vi "Pod Health Status.vi"(7 "Pod Health Configuration":T1={"Power"={"Batt. Current Max (A)"=400.0, " Batt. Current Min (A)"=200.0, "Batt. Voltage Min (V)"=11.5, "Batt. Voltage Max (V)"=13.0, "Brake Current Max (A)"=1.5, " Brake Current Min (A)"=1.3, "Brake Voltage Min (V)"=23.0, "Brake Voltage Max (V)"=25.0}, "Pressure"={"Tank Max (PSI)"=3000.0, "Tank Min (PSI)"=2000.0, "Utility Max (PSI)"=350.0, "Utility Min (PSI)"=250.0, "Brake Max (PSI)"=250.0, "Brake Min (PSI)"=150.0, "Levitation Max (PSI)"=55.0, "Levitation Min (PSI)"=45.0}, "Position"={"Lev. Min (mm)"=35.0, "Lev. Max (mm)"=75.0}}, 10 "Telemetry":T2 {"Brake Pressure (PSI)" scale=0.0..1000.0; "Maglock 4 (mm)" scale=0.0..15.0; "Maglock 3 (mm)" scale=0.0..15.0; "Maglock 2 (mm)" scale=0.0..15.0; "Maglock 1 (mm)" scale=0.0..15.0; "ToF 4 (mm)" scale=0.0..100.0; "ToF 3 (mm)" scale=0.0..100.0; "ToF 2 (mm)" scale=0.0..100.0; "ToF 1 (mm)" scale=0.0..100.0; "Levitation Pressure (PSI)" scale=0.0..1000.0; "Utility Pressure (PSI)" scale=0.0..1000.0; "Tank Pressure (PSI)" scale=0.0..1000.0; "Brake Voltage (V)" scale=0.0..15.0; "Battery Voltage (V)" scale=0.0..15.0; "Brake Current (A)" scale=0.0..500.0; "Battery Current (A)" scale=0.0..500.0}) -> (2 "Pod Health":T3)   [LabVIEW 2018]
uses:
  Type Defs/PodHealth.ctl
  Type Defs/prettyTelemetry.ctl
  Type Defs/PodHealthConfig.ctl
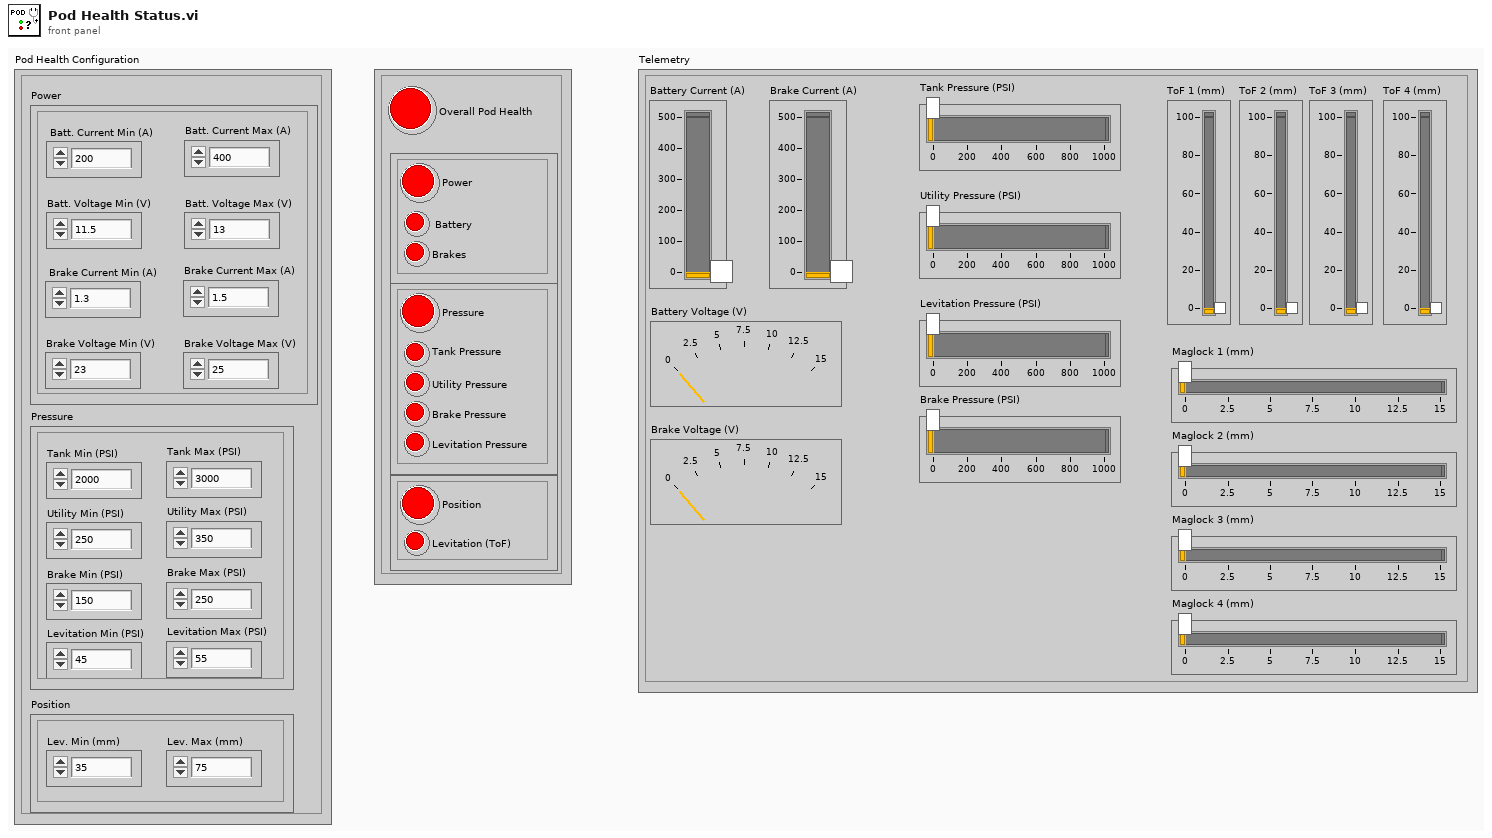
[diagram p1: front panel]
types:
  T1 = typedef "PodHealthConfig.ctl" = cluster{"Power":cluster{"Batt. Current Max (A)":dbl, " Batt. Current Min (A)":dbl, "Batt. Voltage Min (V)":dbl, "Batt. Voltage Max (V)":dbl, "Brake Current Max (A)":dbl, " Brake Current Min (A)":dbl, "Brake Voltage Min (V)":dbl, "Brake Voltage Max (V)":dbl}, "Pressure":cluster{"Tank Max (PSI)":dbl, "Tank Min (PSI)":dbl, "Utility Max (PSI)":dbl, "Utility Min (PSI)":dbl, "Brake Max (PSI)":dbl, "Brake Min (PSI)":dbl, "Levitation Max (PSI)":dbl, "Levitation Min (PSI)":dbl}, "Position":cluster{"Lev. Min (mm)":dbl, "Lev. Max (mm)":dbl}}
  T2 = typedef "prettyTelemetry.ctl" = cluster{"Battery Current (A)":dbl, "Brake Current (A)":dbl, "Battery Voltage (V)":dbl, "Brake Voltage (V)":dbl, "Tank Pressure (PSI)":dbl, "Utility Pressure (PSI)":dbl, "Levitation Pressure (PSI)":dbl, "Brake Pressure (PSI)":dbl, "ToF 1 (mm)":dbl, "ToF 2 (mm)":dbl, "ToF 3 (mm)":dbl, "ToF 4 (mm)":dbl, "Maglock 1 (mm)":dbl, "Maglock 2 (mm)":dbl, "Maglock 3 (mm)":dbl, "Maglock 4 (mm)":dbl}
  T3 = typedef "PodHealth.ctl" = cluster{"Overall Pod Health":bool, "Power":cluster{"Power":bool, " Battery":bool, "Brakes":bool}, "Pressure":cluster{"Pressure":bool, "Tank Pressure":bool, "Utility Pressure":bool, "Brake Pressure":bool, "Levitation Pressure":bool}, "Position":cluster{"Position":bool, "Levitation (ToF)":bool}}
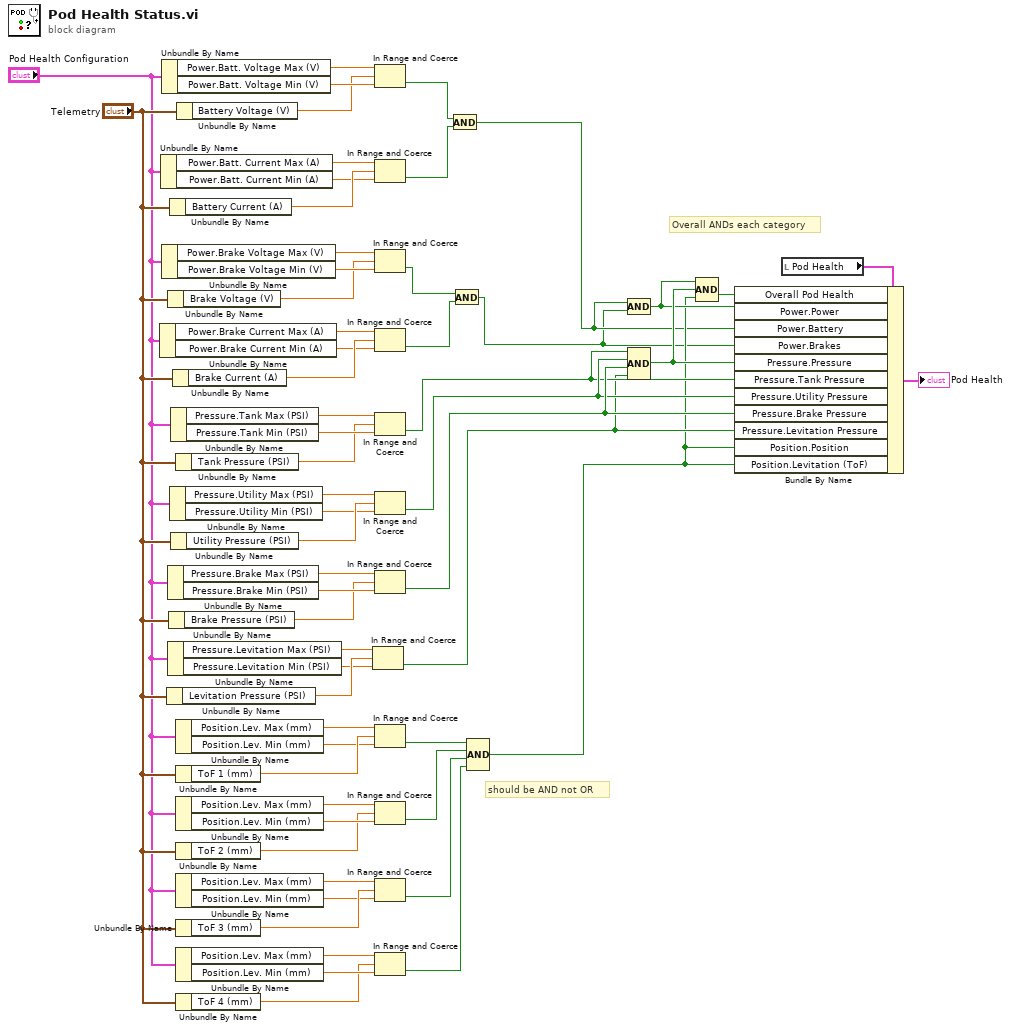
[diagram p0: block diagram]
diagram:
  # "should be AND not OR"
  # "Overall ANDs each category"
  n1 = Unbundle By Name("Pod Health Configuration") -> ("Power.Brake Current Max (A)"=w45:dbl, "Power.Brake Current Min (A)"=w46:dbl)
  n2 = Unbundle By Name("Pod Health Configuration") -> ("Power.Batt. Current Max (A)"=w53:dbl, "Power.Batt. Current Min (A)"=w54:dbl)
  n3 = Unbundle By Name("Pod Health Configuration") -> ("Power.Batt. Voltage Max (V)"=w58:dbl, "Power.Batt. Voltage Min (V)"=w57:dbl)
  n4 = Unbundle By Name("Pod Health Configuration") -> ("Power.Brake Voltage Max (V)"=w50:dbl, "Power.Brake Voltage Min (V)"=w49:dbl)
  n5 = Unbundle By Name("Telemetry") -> ("Levitation Pressure (PSI)"=w13:dbl)
  n6 = Unbundle By Name("Telemetry") -> ("Brake Voltage (V)"=w48:dbl)
  n7 = Unbundle By Name("Pod Health Configuration") -> ("Pressure.Brake Max (PSI)"=w38:dbl, "Pressure.Brake Min (PSI)"=w37:dbl)
  n8 = Unbundle By Name("Pod Health Configuration") -> ("Pressure.Levitation Max (PSI)"=w11:dbl, "Pressure.Levitation Min (PSI)"=w12:dbl)
  n9 = Unbundle By Name("Telemetry") -> ("Brake Pressure (PSI)"=w36:dbl)
  n10 = Unbundle By Name("Telemetry") -> ("Battery Current (A)"=w55:dbl)
  n11 = Unbundle By Name("Pod Health Configuration") -> ("Pressure.Utility Max (PSI)"=w39:dbl, "Pressure.Utility Min (PSI)"=w40:dbl)
  n12 = Unbundle By Name("Pod Health Configuration") -> ("Pressure.Tank Max (PSI)"=w44:dbl, "Pressure.Tank Min (PSI)"=w43:dbl)
  n13 = Unbundle By Name("Telemetry") -> ("Utility Pressure (PSI)"=w41:dbl)
  n14 = Unbundle By Name("Telemetry") -> ("Brake Current (A)"=w47:dbl)
  n15 = Unbundle By Name("Telemetry") -> ("Tank Pressure (PSI)"=w42:dbl)
  n16 = Unbundle By Name("Pod Health Configuration") -> ("Position.Lev. Max (mm)"=w33:dbl, "Position.Lev. Min (mm)"=w34:dbl)
  n17 = Unbundle By Name("Telemetry") -> ("ToF 1 (mm)"=w35:dbl)
  n18 = Unbundle By Name("Pod Health Configuration") -> ("Position.Lev. Max (mm)"=w32:dbl, "Position.Lev. Min (mm)"=w31:dbl)
  n19 = Unbundle By Name("Telemetry") -> ("ToF 2 (mm)"=w30:dbl)
  n20 = Unbundle By Name("Pod Health Configuration") -> ("Position.Lev. Max (mm)"=w27:dbl, "Position.Lev. Min (mm)"=w28:dbl)
  n21 = Unbundle By Name("Telemetry") -> ("ToF 3 (mm)"=w29:dbl)
  n22 = Unbundle By Name("Pod Health Configuration") -> ("Position.Lev. Max (mm)"=w26:dbl, "Position.Lev. Min (mm)"=w25:dbl)
  n23 = Unbundle By Name("Telemetry") -> ("ToF 4 (mm)"=w24:dbl)
  n24 = Unbundle By Name("Telemetry") -> ("Battery Voltage (V)"=w56:dbl)
  n25 = In Range and Coerce(upper limit=w11, x=w13, lower limit=w12) -> (In Range?=w10:bool)  [unwired: 1 out]
  n26 = In Range and Coerce(upper limit=w58, x=w56, lower limit=w57) -> (In Range?=w6:bool)  [unwired: 1 out]
  n27 = In Range and Coerce(upper limit=w53, x=w55, lower limit=w54) -> (In Range?=w5:bool)  [unwired: 1 out]
  n28 = In Range and Coerce(upper limit=w50, x=w48, lower limit=w49) -> (In Range?=w4:bool)  [unwired: 1 out]
  n29 = In Range and Coerce(upper limit=w45, x=w47, lower limit=w46) -> (In Range?=w3:bool)  [unwired: 1 out]
  n30 = In Range and Coerce(upper limit=w44, x=w42, lower limit=w43) -> (In Range?=w17:bool)  [unwired: 1 out]
  n31 = In Range and Coerce(upper limit=w39, x=w41, lower limit=w40) -> (In Range?=w18:bool)  [unwired: 1 out]
  n32 = In Range and Coerce(upper limit=w38, x=w36, lower limit=w37) -> (In Range?=w19:bool)  [unwired: 1 out]
  n33 = In Range and Coerce(upper limit=w33, x=w35, lower limit=w34) -> (In Range?=w23:bool)  [unwired: 1 out]
  n34 = In Range and Coerce(upper limit=w32, x=w30, lower limit=w31) -> (In Range?=w20:bool)  [unwired: 1 out]
  n35 = In Range and Coerce(upper limit=w27, x=w29, lower limit=w28) -> (In Range?=w21:bool)  [unwired: 1 out]
  n36 = In Range and Coerce(upper limit=w26, x=w24, lower limit=w25) -> (In Range?=w22:bool)  [unwired: 1 out]
  n37 = And(x=w6, y=w5) -> (x .and. y?=w2:bool)
  n38 = And(x=w4, y=w3) -> (x .and. y?=w1:bool)
  n39 = Compound Arithmetic op=AND(w23, w20, w21, w22) -> (w7:bool)
  n40 = Compound Arithmetic op=AND(w2, w1) -> (w14:bool)
  n41 = Compound Arithmetic op=AND(w17, w18, w19, w10) -> (w15:bool)
  n42 = Compound Arithmetic op=AND(w14, w15, w7) -> (w16:bool)
  n43 = local read "Pod Health"() -> (w52:T3)
  n44 = Bundle By Name(cluster=w52, "Overall Pod Health"=w16, "Power.Power"=w14, "Power.Battery"=w2, "Power.Brakes"=w1, "Pressure.Pressure"=w15, "Pressure.Tank Pressure"=w17, "Pressure.Utility Pressure"=w18, "Pressure.Brake Pressure"=w19, "Pressure.Levitation Pressure"=w10, "Position.Position"=w7, "Position.Levitation (ToF)"=w7) -> (→"Pod Health":T3)
